vi "Sequence Start set(Templet).vi"(7 "Channel  (1: CH1)":u16(ring)=1 items=["CH1"=1, "CH2"=2, "CH3"=3, "CH4"=4], 8 "error in (no error)":errorcluster, 10 "Start":u32, 11 "VISA resource in":refnum<visa-resource-name>) -> (0 "error out":errorcluster, 3 "VISA resource name out":refnum<visa-resource-name>)   [LabVIEW 2020, in "GPP.lvlib"]
uses:
  GPP.lvlib
  Function/VISA_COMMON.ctl
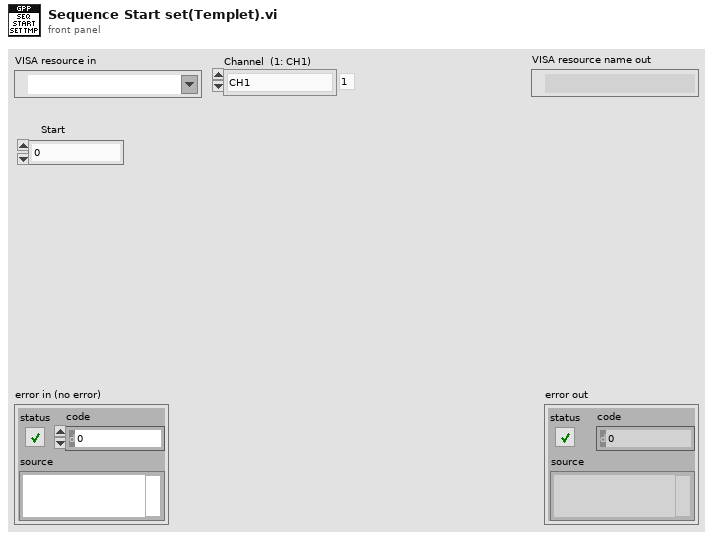
[diagram p1: front panel]
types:
  T1 = typedef "GPP.lvlib/VISA_COMMON.ctl" = enum16{"Initial", "Write CMD", "Read Result", "Read History", "Close"}
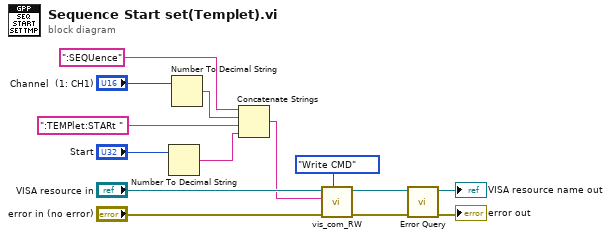
[diagram p0: block diagram]
diagram:
  n1 = Number To Decimal String(number="Start") -> (decimal integer string=w12:string)  [unwired: 1 in]
  n2 = Number To Decimal String(number="Channel  (1: CH1)") -> (decimal integer string=w14:string)  [unwired: 1 in]
  n3 = Concatenate Strings(":SEQUence", w14, ":TEMPlet:STARt ", w12) -> (w3:string)
  n4 = call "vis_com_RW.vi"("Funciton"=VISA_COMMON."Write CMD", "error in (no error)"="error in (no error)", "CMD String"=w3, "VISA resource in"="VISA resource in") -> ("error out"=w9:errorcluster, "VISA resource out"=w10:refnum<visa-resource-name>)  [unwired: 5 in, 1 out]
  n5 = call "Error Query.vi"("error in (no error)"=w9, "VISA resource name"=w10) -> ("error out"=→"error out":errorcluster, "VISA resource name out"=→"VISA resource name out":refnum<visa-resource-name>)  [unwired: 6 in, 2 out]
